vi "worksheet insert image opt.vi"(6 "options":T1, 7 "filename":string, 8 "error in (no error)":errorcluster, 9 "col":u16, 10 "row":u32, 11 "worksheet":u32) -> (0 "error out":errorcluster, 3 "function return":u32(ring), 4 "options out":T1)   [LabVIEW 2015, in "xlsxwriter.lvlib"]
doc: "lxw_error worksheet_insert_image_opt(lxw_worksheet worksheet, lxw_row_t row, lxw_col_t col, const char *filename, lxw_image_options *options);"
uses:
  xlsxwriter.lvlib
  xlsxwriter.dll
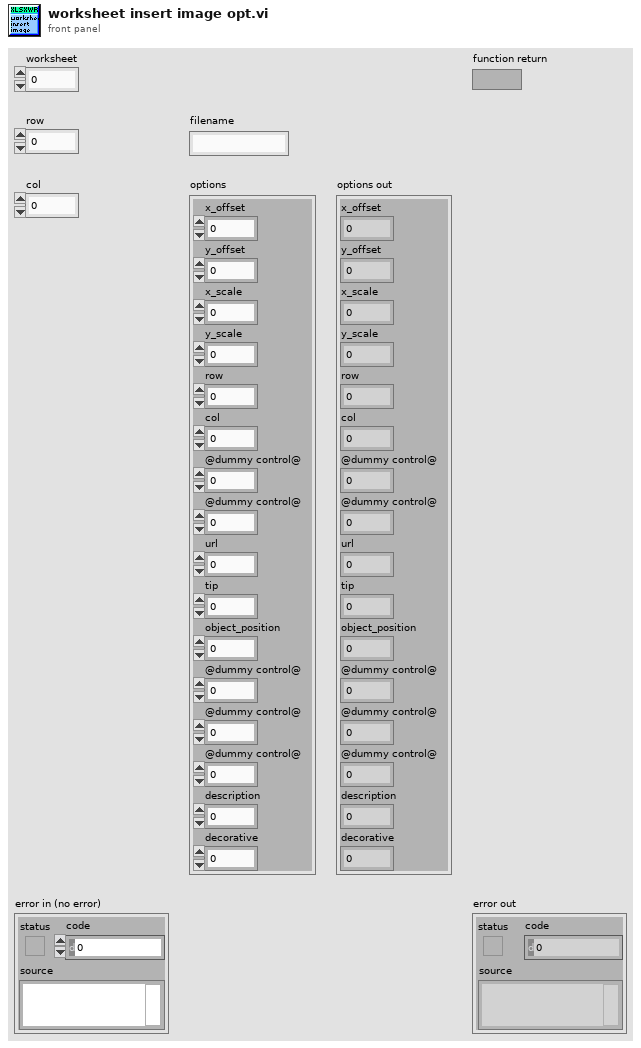
[diagram p1: front panel]
types:
  T1 = cluster{"x_offset":i32, "y_offset":i32, "x_scale":dbl, "y_scale":dbl, "row":u32, "col":u16, "@dummy control@":i8, "@dummy control@":i8, "url":u32, "tip":u32, "object_position":u8, "@dummy control@":i8, "@dummy control@":i8, "@dummy control@":i8, "description":u32, "decorative":u32}
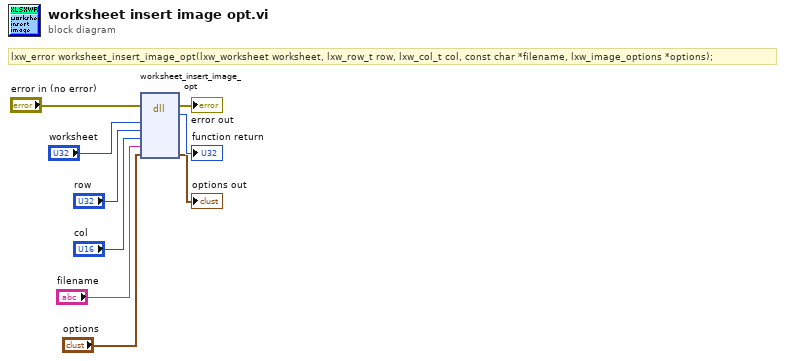
[diagram p0: block diagram]
diagram:
  # "lxw_error worksheet_insert_image_opt(lxw_worksheet worksheet, lxw_row_t row, lxw_col_t col, const char *filename, lxw_image_options *options);"
  n1 = dll-call lib="C:/Users/WDAGUtilityAccount/Desktop/lv_vis_added_cell/xlsxwriter.*" fn="worksheet_insert_image_opt"(error in="error in (no error)", "worksheet"="worksheet", "row"="row", "col"="col", "filename"="filename", "options"="options") -> (error out=→"error out":errorcluster, →"function return":u32, "options"=→"options out":T1)  [unwired: 6 in, 1 out]
